vi "UT_UserEventHandler_Main.vi"(8 "error in (no error)":errorcluster) -> (0 "error out":errorcluster)   [LabVIEW 2016, in "UT_UserEventHandler.lvlib"]
doc: "Collection of tests for the UserEventHandler class."
uses:
  UT_UserEventHandler.lvlib
  <vilib>/addons/_JKI Toolkits/Caraya/classes/Test/Test.lvclass
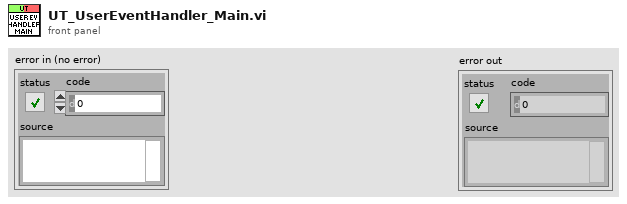
[diagram p1: front panel]
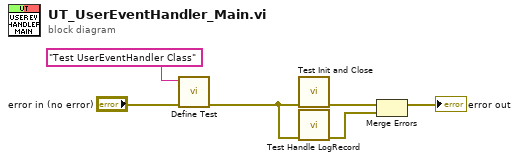
[diagram p0: block diagram]
diagram:
  n1 = call <vilib>:"Define Test.vi"("error in (no error)"="error in (no error)", "Label (VI Title)"="Test UserEventHandler Class") -> ("error out"=w4:errorcluster)  [unwired: 9 in]
  n2 = call "Test Init and Close.vi"("error in (no error)"=w4) -> ("error out"=w3:errorcluster)  [unwired: 10 in]
  n3 = call "Test Handle LogRecord.vi"("error in (no error)"=w4) -> ("error out"=w2:errorcluster)  [unwired: 10 in]
  n4 = Merge Errors(w3, w2) -> (→"error out":errorcluster)
